vi "initialize.vi"(8 "error in (no error)":errorcluster, 11 "LakeShore336 in":refnum<class "Lakeshore_336.lvclass">) -> (0 "error out":errorcluster, 1 "String Output":string, 2 "initialized?":bool, 3 "LakeShore336 out":refnum<class "Lakeshore_336.lvclass">)   [LabVIEW 2017, in "Lakeshore_336.lvclass"]
doc: "initializes an instrument; this method is going to be replaced by the same method of the child objects"
uses:
  Lakeshore_336.lvclass
  instrument.lvclass
  Drivers/Lake Shore 336/Lake Shore 336.lvlib
panel:
  in  "Serial Configuration":T1={"Baud Rate"=57600, "Parity"=1, "Data Bits"=7, "Stop Bits"=10, "Flow Control"=0} {"Flow Control" items=["None", "XON/XOFF", "RTS/CTS", "XON/XOFF & RTS/CTS", "DTR/DSR", "XON/XOFF & DTR/DSR"]; "Stop Bits" items=["1.0"=10, "1.5"=15, "2.0"=20]; "Data Bits" items=["7"=7, "8"=8]; "Parity" items=["None", "Odd", "Even", "Mark", "Space"]; "Baud Rate" items=["300"=300, "600"=600, "1200"=1200, "2400"=2400, "4800"=4800, "9600"=9600, "19200"=19200, "38400"=38400, "57600"=57600]}
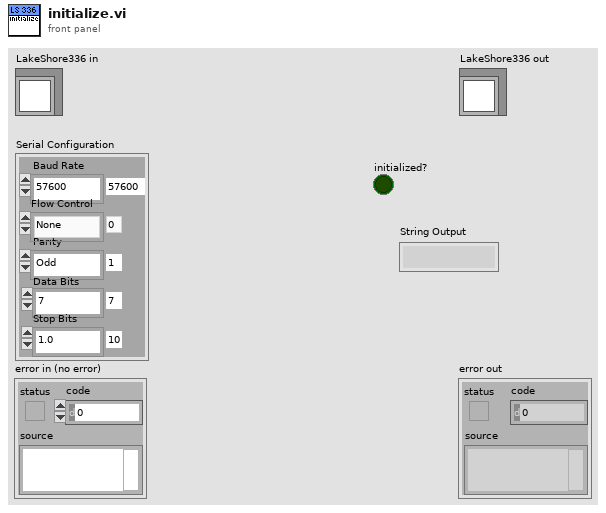
[diagram p1: front panel]
types:
  T1 = cluster{"Baud Rate":u32, "Parity":u16, "Data Bits":u16, "Stop Bits":u16, "Flow Control":u16}
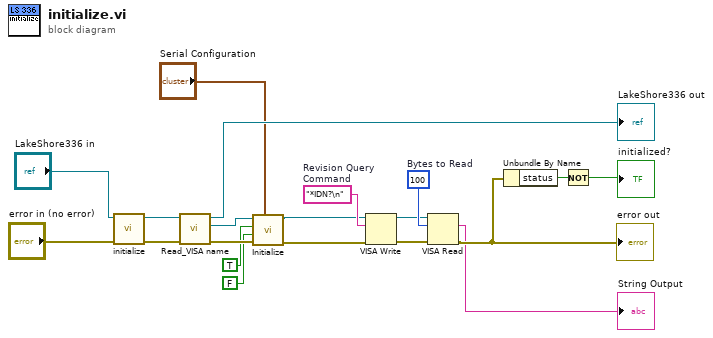
[diagram p0: block diagram]
diagram:
  w5 = "*IDN?\n"  # Revision Query Command
  w8 = u32 100  # Bytes to Read
  n1 = call-parent "initialize.vi"("error in (no error)"="error in (no error)", "instrument in"="LakeShore336 in") -> ("error out"=w17:errorcluster, "instrument out"=w18:refnum<class "Lakeshore_336.lvclass">)  [unwired: 6 in, 2 out]
  n2 = call-dynamic "Read_VISA name.vi"("error in (no error)"=w17, "instrument in"=w18) -> ("error out"=w15:errorcluster, "VISA resource name"=w14:refnum<visa-resource-name>, "instrument out"=→"LakeShore336 out":refnum<class "Lakeshore_336.lvclass">)  [unwired: 7 in]
  n3 = call "Initialize.vi"("Serial Configuration"="Serial Configuration", "error in (no error)"=w15, "Reset (True)"=FALSE, "ID Query (True)"=TRUE, "VISA resource name"=w14) -> ("error out"=w3:errorcluster, "VISA resource name out"=w4:refnum<visa-resource-name>)  [unwired: 5 in]
  n4 = VISA Write(VISA resource name=w4, write buffer=w5, error in (no error)=w3) -> (VISA resource name out=w7:refnum<visa-resource-name>, error out=w6:errorcluster)  [unwired: 1 out]
  n5 = VISA Read(VISA resource name=w7, byte count=w8, error in (no error)=w6) -> (read buffer=→"String Output":string, error out=w2:errorcluster)  [unwired: 2 out]
  "error out" <- w2
  n6 = Unbundle By Name(w2) -> ("status"=w10:bool)
  n7 = Not(x=w10) -> (.not. x?=→"initialized?":bool)
